vi "Receive Vision Packet.vi"(11 "connection ID":refnum<k16>) -> ()   [LabVIEW 2014]
uses:
  2015 Crabby Dashboard Project/Vision/Vision Tote Data.ctl
  Common Code/Vision Packet.ctl
  Robot Global Data.vi
  Common Code/Elevator Object Type.ctl
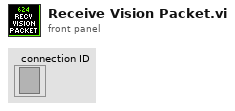
[diagram p1: front panel]
types:
  T1 = typedef "Vision Packet.ctl" = cluster{"Vision Tote":T2, "Gyro Value":dbl, "Elevator Obj Found?":bool, "Elevator Obj":T3}
  T2 = typedef "Vision Tote Data.ctl" = cluster{"Left _|":cluster{"Bounding box":cluster{"left":dbl, "top":dbl, "right":dbl, "bottom":dbl}, "Aspect Ratio":dbl, "Area Score":dbl, "X Mask":dbl, "Y Mask":dbl, "Ell":bool}, "Right |_":cluster{"Bounding box":cluster{"left":dbl, "top":dbl, "right":dbl, "bottom":dbl}, "Aspect Ratio":dbl, "Area Score":dbl, "X Mask":dbl, "Y Mask":dbl, "Ell":bool}, "Center X":dbl, "Center Y":dbl, "Angle Offset":dbl}
  T3 = typedef "Elevator Object Type.ctl" = enum16{"Grey Tote", "Yellow Tote", "Trash Can"}
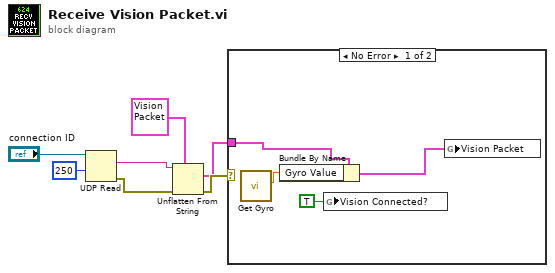
[diagram p0: block diagram]
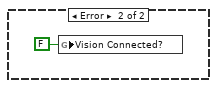
[diagram p2: hidden frame]
diagram:
  n1 = UDP Read(connection ID="connection ID", timeout ms (25000)=250) -> (data out=w6:string, error out=w1:errorcluster)  [unwired: 2 in, 3 out]
  n2 = Unflatten From String(type=T1 {"Vision Tote"={"Left _|"={"Bounding box"={"left"=0.0, "top"=0.0, "right"=0.0, "bottom"=0.0}, "Aspect Ratio"=0.0, "Area Score"=0.0, "X Mask"=0.0, "Y Mask"=0.0, "Ell"=FALSE}, "Right |_"={"Bounding box"={"left"=0.0, "top"=0.0, "right"=0.0, "bottom"=0.0}, "Aspect Ratio"=0.0, "Area Score"=0.0, "X Mask"=0.0, "Y Mask"=0.0, "Ell"=FALSE}, "Center X"=0.0, "Center Y"=0.0, "Angle Offset"=0.0}, "Gyro Value"=0.0, "Elevator Obj Found?"=FALSE, "Elevator Obj"=enum."Grey Tote"} ("Vision Packet"), binary string=w6, error in (no error)=w1) -> (value=w2:T1, error out=w3:errorcluster)  [unwired: 2 in, 1 out]
  n3 = case shown="No Error" w3 {
    tunnel: w2 -> [w10 _]
    frame No Error {
      n4 = call "Get Gyro.vi"() -> ("Angle"=w9:dbl)  [unwired: 11 in]
      n5 = Bundle By Name(cluster=w10, "Gyro Value"=w9) -> (w8:T1)
      n6 = global write "Robot Global Data.vi" "Vision Connected?"(TRUE ("Vision Connected?")) -> ()
      n7 = global write "Robot Global Data.vi" "Vision Packet"(w8) -> ()
    }
    frame Error {
      n8 = global write "Robot Global Data.vi" "Vision Connected?"(FALSE ("Vision Connected?")) -> ()
    }
  }
